vi "Find Object Item Locations by Names.vi"(5 "Insertion point if not found":bool, 6 "Only return first found":bool, 7 "Item Names <JSON>":string[](array[string]), 8 "error in (no error)":errorcluster, 10 "Object Offset":i32, 11 "JSON":string) -> (0 "error out":errorcluster, 1 "Items":T1[](array[typedef]))   [LabVIEW 2024, in "JSONtext.lvlib"]
uses:
  JSONtext.lvlib
  Found Items.ctl
  Parsing State.ctl
  Comma Needed for Insert.ctl
  Advance past Line Ending.vi
  Advance past String.vi
  Advance past Number.vi
  Advance past Array.vi
  Advance past Object.vi
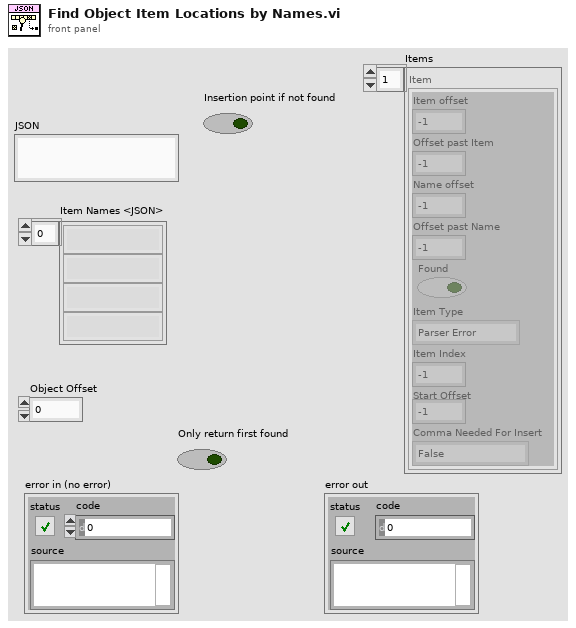
[diagram p1: front panel]
types:
  T1 = typedef "JSONtext.lvlib/Found Items.ctl" = cluster{"Item offset":i32, "Offset past Item":i32, "Name offset":i32, "Offset past Name":i32, "Found":bool, "Item Type":T2, "Item Index":i32, "Start Offset":i32, "Comma Needed For Insert":T3}
  T2 = typedef "JSONtext.lvlib/Parsing State.ctl" = enum16{"Parser Error", "Object", "Array", "String", "Number/Other", "Leading Whitespace", "Object end", "Array end", "Value end"}
  T3 = typedef "JSONtext.lvlib/Comma Needed for Insert.ctl" = enum8{"False", "True", "Following"}
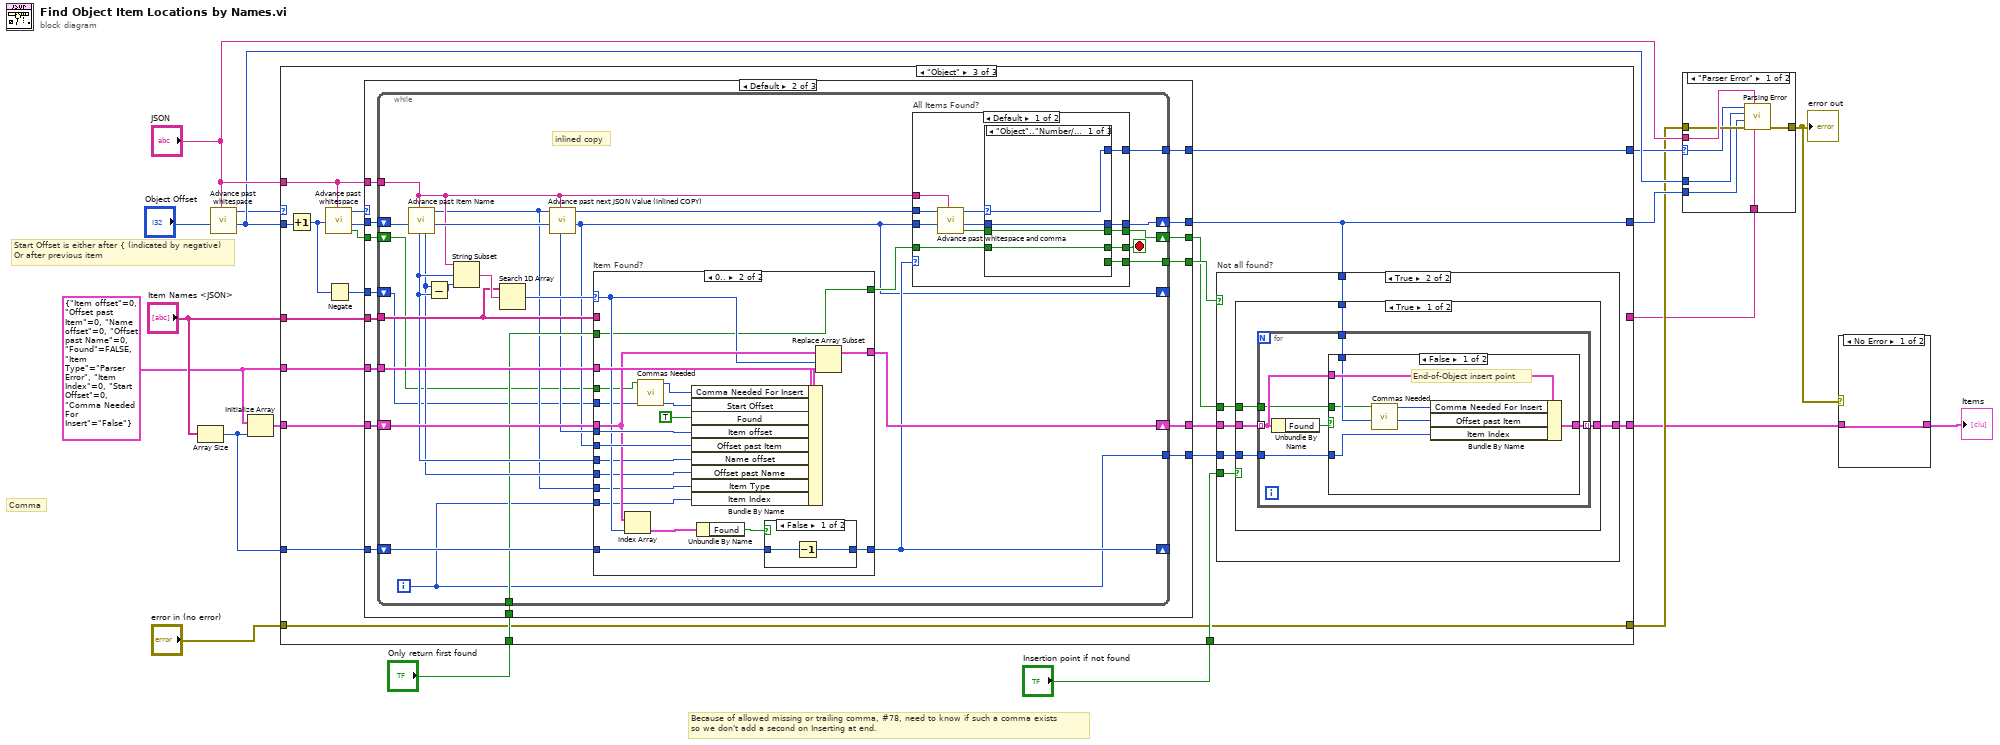
[diagram p0: block diagram]
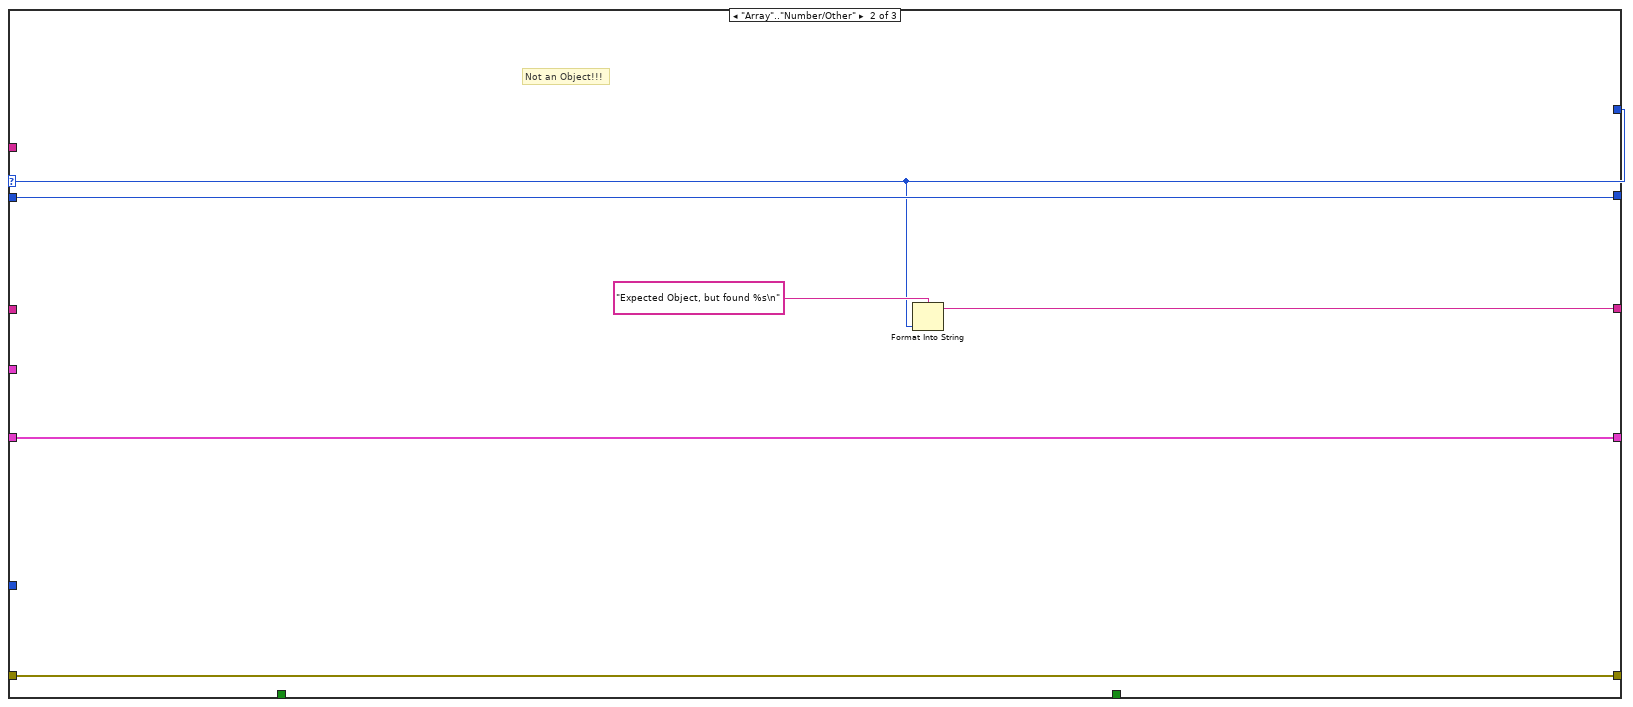
[diagram p3: hidden frame]
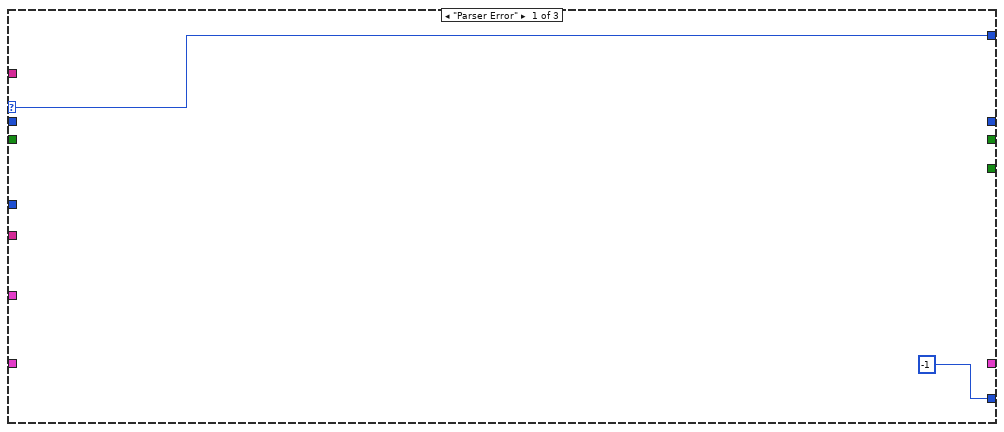
[diagram p4: hidden frame]
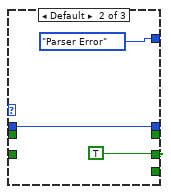
[diagram p7: hidden frame]
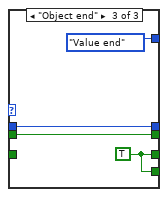
[diagram p8: hidden frame]
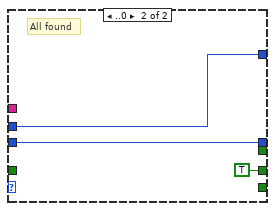
[diagram p9: hidden frame]
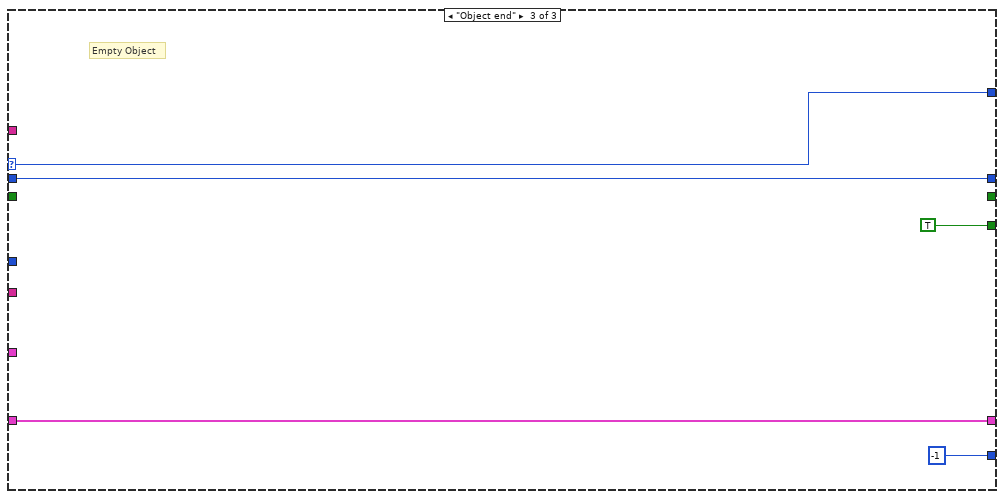
[diagram p10: hidden frame]
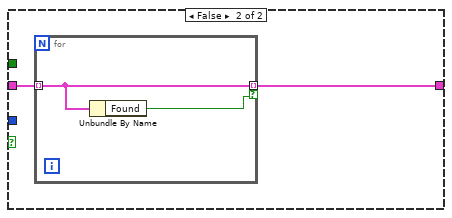
[diagram p13: hidden frame]
diagram:
  w15 = T1 {"Item offset"=0, "Offset past Item"=0, "Name offset"=0, "Offset past Name"=0, "Found"=FALSE, "Item Type"=enum."Parser Error", "Item Index"=0, "Start Offset"=0, "Comma Needed For Insert"=enum."False"}
  # "Because of allowed missing or trailing comma, #78, need to know if such a comma exists \nso we don't add a second on Inserting at end."
  # "Comma"
  # "Start Offset is either after { (indicated by negative)\nOr after previous item"
  n1 = Array Size(array="Item Names <JSON>") -> (size(s)=w14:i32)
  n2 = call "Advance past whitespace.vi"("JSON"="JSON", "Offset"="Object Offset") -> ("Offset of first non-whitespace"=w11:i32, "Parser State"=w10:T2)  [unwired: 7 in, 1 out]
  n3 = Initialize Array(w15, w14) -> (w16:T1[])
  n4 = case shown="\"Object\"" w10 {
    selector: w10 -> [w19 w24 _]
    tunnel: "Item Names <JSON>" -> [_ _ w49]
    tunnel: w16 -> [w22 w28 w48]
    tunnel: w15 -> [_ _ w47]
    tunnel: w14 -> [_ _ w46]
    tunnel: [w22 w28 w43] -> w2
    tunnel: "JSON" -> [_ _ w37]
    tunnel: [w20 w26 w42] -> w12
    tunnel: w11 -> [w20 w26 w33]
    tunnel: [w19 w24 w41] -> w9
    tunnel: "Only return first found" -> [_ _ w40]
    tunnel: "Insertion point if not found" -> [_ _ w39]
    tunnel: "error in (no error)" -> [w21 w27 w38]
    tunnel: [w21 w27 w38] -> w5
    tunnel: [_ w23 _] -> w1
    frame "Parser Error", Default {
      # "Not an Object!!!"
    }
    frame "Array".."Number/Other" {
      # "Not an Object!!!"
      n5 = Format Into String(format string="Expected Object, but found %s\n", w24) -> (resulting string=w23:string)  [unwired: 2 in, 1 out]
    }
    frame "Object" {
      n6 = Increment(x=w33) -> (x+1=w32:i32)
      n7 = call "Advance past whitespace.vi"("JSON"=w37, "Offset"=w32) -> ("Comma Not Found"=w29:bool, "Offset of first non-whitespace"=w36:i32, "Parser State"=w35:T2)  [unwired: 7 in]
      n8 = Negate(x=w32) -> (-x=w31:i32)
      n9 = case shown="Default" w35 {
        selector: w35 -> [w51 _ w149]
        tunnel: w36 -> [_ w66 w148]
        tunnel: w49 -> [_ w65 _]
        tunnel: w48 -> [_ w64 w147]
        tunnel: w47 -> [_ w63 _]
        tunnel: w46 -> [_ w62 _]
        tunnel: [_ w61 w147] -> w45
        tunnel: [_ w60 TRUE] -> w44
        tunnel: w37 -> [_ w59 _]
        tunnel: [_ w58 w148] -> w42
        tunnel: [w51 w57 w149] -> w41
        tunnel: w40 -> [_ w56 _]
        tunnel: [-1 w55 -1] -> w34
        tunnel: w31 -> [_ w54 _]
        tunnel: [_ w53 _] -> w30
        tunnel: w29 -> [_ w52 _]
        frame "Parser Error" {
        }
        frame Default {
          n10 = while {
            shift-right: [w94] -> w58
            shift-left: w66 -> [w91]
            tunnel: w59 -> [w88]
            tunnel: [w92] -> w57
            tunnel: w65 -> [w83]
            tunnel: w63 -> [w85]
            shift-right: [w81] -> w61
            shift-left: w64 -> [w82]
            shift-right: [w79] -> _
            shift-left: w62 -> [w80]
            tunnel: [w78] -> w60
            tunnel: w56 -> [w75]
            tunnel: [w71] -> w55
            shift-right: [w70] -> _
            shift-left: w54 -> [w69]
            shift-right: [w68] -> w53
            shift-left: w52 -> [w67]
            i -> [w71]
            stop <- w93 stop-if-true
            # "inlined copy"
            n11 = call "Advance past Item Name.vi"("JSON"=w88, "Offset"=w91) -> ("Offset past colon"=w89:i32, "State"=w72:T2, "Offset past Name"=w76:i32, "Name start out"=w77:i32)  [unwired: 6 in]
            n12 = Subtract(x=w76, y=w77) -> (x-y=w87:i32)
            n13 = String Subset(string=w88, offset (0)=w77, length (rest)=w87) -> (substring=w86:string)
            n14 = Search 1D Array(1D array=w83, element=w86) -> (index of element=w84:i32)  [unwired: 1 in]
            n15 = call "Advance past next JSON Value (inlined COPY).vi"("JSON"=w88, "Offset"=w89, "State"=w72) -> ("Offset"=w70:i32, "State"=w90:T2, "Value start"=w73:i32)  [unwired: 4 in, 2 out]
            n16 = case "Item Found?" shown="0.." w84 {
              selector: w84 -> [_ w110]
              tunnel: w85 -> [_ w116]
              tunnel: w73 -> [_ w114]
              tunnel: w70 -> [_ w113]
              tunnel: w83 -> [_ _]
              tunnel: w82 -> [w96 w111]
              tunnel: [w96 w109] -> w81
              tunnel: w80 -> [w95 w106]
              tunnel: [w95 w105] -> w79
              tunnel: w77 -> [_ w104]
              tunnel: w76 -> [_ w103]
              tunnel: w75 -> [_ w102]
              tunnel: [_ w102] -> w74
              tunnel: w72 -> [_ w101]
              tunnel: w71 -> [_ w100]
              tunnel: w69 -> [_ w99]
              tunnel: w67 -> [_ w97]
              frame Default {
              }
              frame 0.. {
                n17 = Index Array(array=w111, index=w110) -> (element=w108:T1)
                n18 = call "Commas Needed.vi"("Comma needed"=w97) -> ("Comma Needed For Insert"=w98:T3)  [unwired: 10 in]
                n19 = Bundle By Name(cluster=w116, "Comma Needed For Insert"=w98, "Start Offset"=w99, "Found"=TRUE, "Item offset"=w114, "Offset past Item"=w113, "Name offset"=w104, "Offset past Name"=w103, "Item Type"=w101, "Item Index"=w100) -> (w112:T1)
                n20 = Unbundle By Name(w108) -> ("Found"=w107:bool)
                n21 = case shown="False" w107 {
                  tunnel: w106 -> [w118 w119]
                  tunnel: [w117 w119] -> w105
                  frame False {
                    n22 = Decrement(x=w118) -> (x-1=w117:i32)
                  }
                  frame True {
                  }
                }
                n23 = Replace Array Subset(array=w111, new element=w112, index=w110) -> (w109:T1[])
              }
            }
            n24 = case "All Items Found?" shown="Default" w79 {
              tunnel: [w130 w144] -> w94
              tunnel: [w129 TRUE] -> w93
              tunnel: [w128 w145] -> w92
              tunnel: w90 -> [w123 w145]
              tunnel: w70 -> [w126 w144]
              tunnel: w88 -> [w127 _]
              tunnel: [w124 _] -> w78
              tunnel: w74 -> [w122 _]
              tunnel: [w120 _] -> w68
              frame Default {
                n25 = call "Advance past whitespace and comma.vi"("JSON"=w127, "Offset"=w126, "State in"=w123) -> ("Comma Not Found"=w121:bool, "Offset past match"=w125:i32, "State"=w131:T2)  [unwired: 6 in]
                n26 = case shown="\"Object\"..\"Number/Other\"" w131 {
                  selector: w131 -> [w133 _ _]
                  tunnel: [w134 TRUE w141] -> w129
                  tunnel: [w133 Parsing_State."Parser Error" Parsing_State."Value end"] -> w128
                  tunnel: w125 -> [w135 w136 w140]
                  tunnel: [w135 w136 w140] -> w130
                  tunnel: [_ _ w141] -> w124
                  tunnel: w122 -> [w134 _ _]
                  tunnel: w121 -> [w132 _ w139]
                  tunnel: [w132 _ w139] -> w120
                  frame "Object".."Number/Other" {
                  }
                  frame Default {
                  }
                  frame "Object end" {
                    w141 = TRUE
                  }
                }
              }
              frame ..0 {
                # "All found"
              }
            }
          }
        }
        frame "Object end" {
          # "Empty Object"
        }
      }
      n27 = case "Not all found?" shown="True" w44 {
        tunnel: w45 -> [w151 w157]
        tunnel: [w151 w156] -> w43
        tunnel: w42 -> [_ w155]
        tunnel: w39 -> [_ w154]
        tunnel: w34 -> [_ w153]
        tunnel: w30 -> [_ w152]
        frame False {
        }
        frame True {
          n28 = case shown="True" w154 {
            tunnel: w157 -> [w163 w178]
            tunnel: [w162 w177] -> w156
            tunnel: w155 -> [w161 _]
            tunnel: w153 -> [w160 _]
            tunnel: w152 -> [w158 _]
            frame True {
              n29 = Increment(x=w160) -> (x+1=w159:i32)
              n30 = for {
                tunnel: w163 -> [w167] mode=indexing
                tunnel: [w168] -> w162 mode=indexing
                tunnel: w161 -> [w166]
                tunnel: w159 -> [w165]
                tunnel: w158 -> [w164]
                n31 = Unbundle By Name(w167) -> ("Found"=w169:bool)
                n32 = case shown="False" w169 {
                  tunnel: [w174 w176] -> w168
                  tunnel: w167 -> [w175 w176]
                  tunnel: w166 -> [w173 _]
                  tunnel: w165 -> [w172 _]
                  tunnel: w164 -> [w170 _]
                  frame False {
                    # "End-of-Object insert point"
                    n33 = call "Commas Needed.vi"("Comma needed"=w170) -> ("Comma Needed For Insert"=w171:T3)  [unwired: 10 in]
                    n34 = Bundle By Name(cluster=w175, "Comma Needed For Insert"=w171, "Offset past Item"=w173, "Item Index"=w172) -> (w174:T1)
                  }
                  frame True {
                  }
                }
              }
            }
            frame False {
              n35 = for {
                tunnel: w178 -> [w180] mode=indexing
                tunnel: [w180] -> w177 mode=indexing if=w179
                n36 = Unbundle By Name(w180) -> ("Found"=w179:bool)
              }
            }
          }
        }
      }
    }
  }
  n37 = case shown="\"Parser Error\"" w9 {
    selector: w9 -> [w182 _]
    tunnel: "JSON" -> [w187 _]
    tunnel: w5 -> [w186 w188]
    tunnel: [w185 w188] -> w4
    tunnel: w11 -> [w184 _]
    tunnel: w12 -> [w183 _]
    tunnel: w1 -> [w181 _]
    frame "Parser Error" {
      n38 = call "Parsing Error.vi"("initial string"=w181, "JSON"=w187, "error in (no error)"=w186, "Offset past match"=w183, "Value start"=w184, "State"=w182) -> ("error out"=w185:errorcluster)  [unwired: 5 in]
    }
    frame Default {
    }
  }
  "error out" <- w4
  n39 = case shown="No Error" w4 {
    tunnel: [w189 _] -> w3
    tunnel: w2 -> [w189 _]
    frame No Error {
    }
    frame Error {
    }
  }
  "Items" <- w3
